vi "加载cRIO.vi"(8 "error in (no error)":errorcluster caption="错误输入（无错误）") -> (0 "error out":errorcluster caption="错误输出")   [LabVIEW 2014]
doc: "该模板用于创建子VI。"
uses:
  glb/glb_data.vi
  <vilib>/Utility/config.llb/NI_LVConfig.lvlib
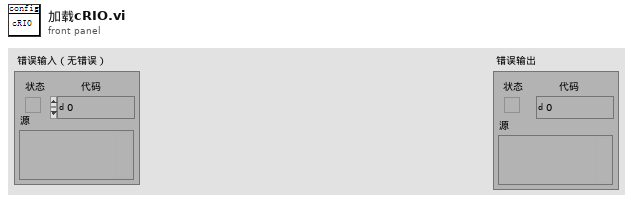
[diagram p1: front panel]
types:
  T1 = typedef "NI_LVConfig.lvlib/Config Data RefNum.ctl" = refnum<k1>
  T2 = cluster{"名称":string, "简称":string, "单位":string, "附加":string[], "类型":enum16{"测试模块", "FPGA", "cRIO", "其他设备", "总体展示"}}
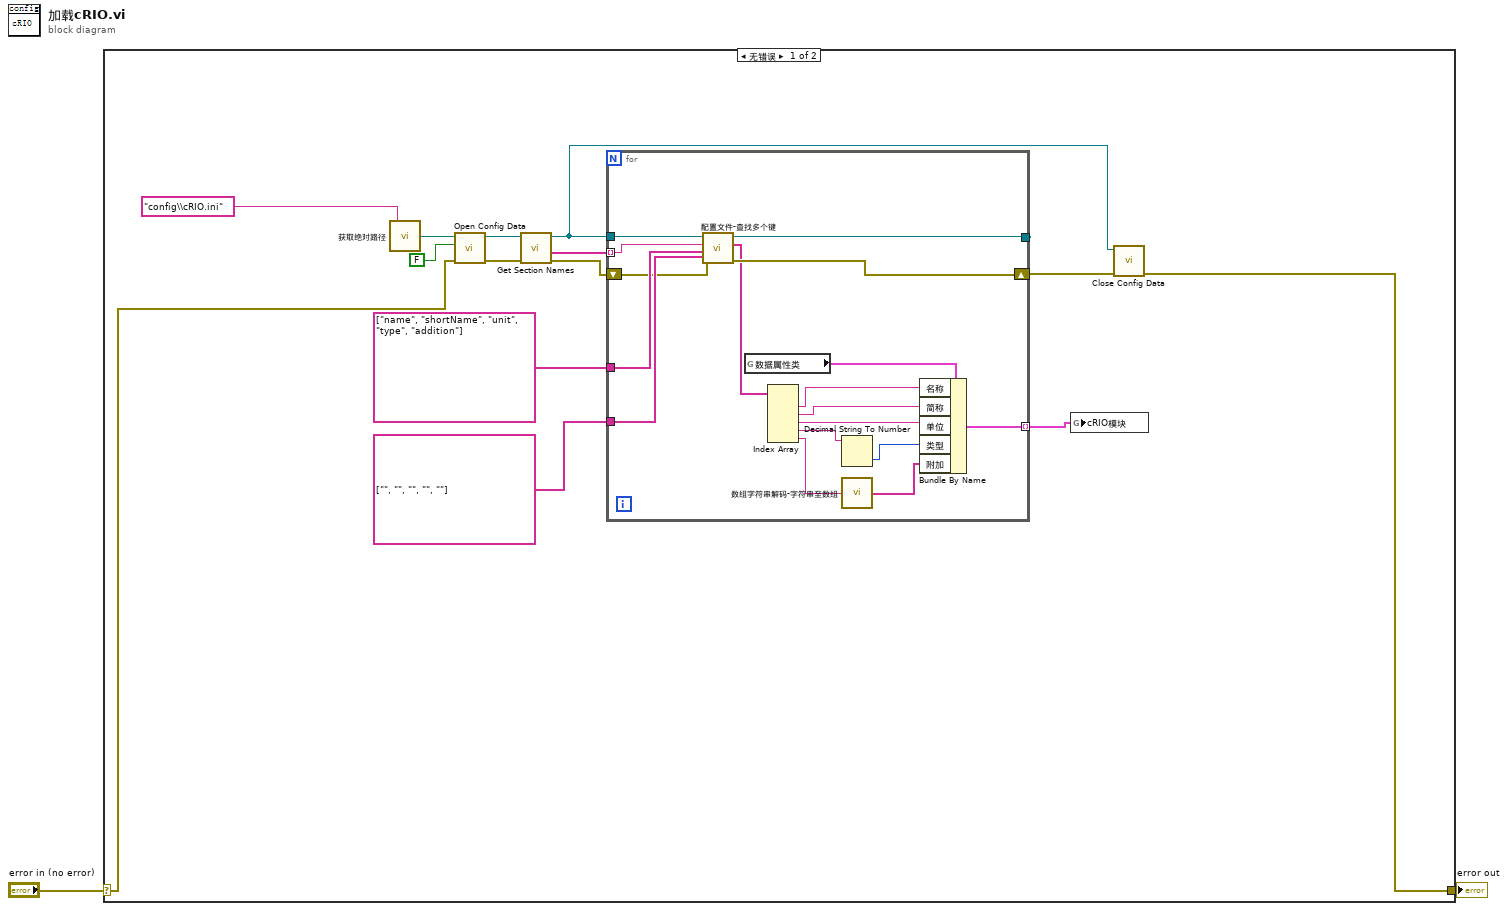
[diagram p0: block diagram]
diagram:
  n1 = case shown="无错误" "error in (no error)" {
    selector: "error in (no error)" -> [w4 w34]
    tunnel: [w16 w34] -> w1
    frame No Error {
      n2 = call "获取绝对路径.vi"("relativePath"="config\\cRIO.ini" ("测试模块配置文件")) -> ("absolutePath"=w15:path)
      n3 = call <vilib>:"Open Config Data.vi"("error in (no error)"=w4, "create file if necessary (T)"=FALSE, "configuration file path"=w15) -> ("error out"=w13:errorcluster, "refnum"=w12:T1)  [unwired: 6 in, 1 out]
      n4 = call <vilib>:"Get Section Names.vi"("error in (no error)"=w13, "refnum"=w12) -> ("error out"=w10:errorcluster, "section names"=w11:string[], "refnum out"=w6:T1)  [unwired: 7 in]
      n5 = for {
        tunnel: w11 -> [w30] mode=indexing
        tunnel: w6 -> [w33]
        shift-right: [w28] -> w7
        shift-left: w10 -> [w29]
        tunnel: string[] ["name", "shortName", "unit", "type", "addition"] -> [w31]
        tunnel: string[] ["", "", "", "", ""] -> [w32]
        tunnel: [w27] -> _
        tunnel: [w17] -> w3 mode=indexing
        n6 = call "配置文件-查找多个键.vi"("默认值"=w32, "错误输入（无错误）"=w29, "键名"=w31, "章名"=w30, "引用句柄输入"=w33) -> ("错误输出"=w28:errorcluster, "查询结果"=w26:string[], "引用句柄输出"=w27:T1)  [unwired: 4 in]
        n7 = global read "类信息.vi" "数据属性类"() -> (w25:T2)
        n8 = Index Array(array=w26) -> (element #1=w24:string, element #2=w23:string, element #3=w22:string, element #4=w21:string, element #5=w19:string)  [unwired: 5 in]
        n9 = Decimal String To Number(string=w21) -> (number=w20:i32)  [unwired: 2 in, 1 out]
        n10 = call "数组字符串解码-字符串至数组.vi"("字符串"=w19) -> ("数组"=w18:string[])  [unwired: 1 in]
        n11 = Bundle By Name(cluster=w25, "名称"=w24, "简称"=w23, "单位"=w22, "类型"=w20, "附加"=w18) -> (w17:T2)
      }
      n12 = global write "glb_data.vi" "cRIO模块"(w3) -> ()
      n13 = call <vilib>:"Close Config Data.vi"("error in (no error)"=w7, "refnum"=w6) -> ("error out"=w16:errorcluster)  [unwired: 8 in, 1 out]
    }
    frame Error {
    }
  }
  "error out" <- w1
